vi "Execute Add Actor Message.vi"(6 "Mouse Position":T1 caption="鼠标位置", 8 "User VI Ref":refnum<vi> caption="用户VI引用", 9 "Menu Item Tag Suffix":string caption="菜单项标签后缀", 10 "Remaining Items":refnum<vi>[](array[refnum]) caption="剩余项", 11 "Affected Items":T2 caption="受影响的项") -> (0 "Fail transaction?":bool caption="操作失败？")   [LabVIEW 2020]
doc: "该VI属于修改LabVIEW快捷菜单部分。这是用户选择快捷菜单时调用的执行VI。该VI执行选中菜单项的操作。"
uses:
  Add Actor Message.ctl
  <vilib>/Utility/miscctls.llb/LVPositionTypeDef.ctl
panel:
  # "除“受影响的项”之外，前面板上的其他所有控件都已锁定，以防被意外编辑。修改控件名称或类型，而不是“受影响的项”簇的元素将使VI无法作为菜单插件使用。\n\n请参考每个控件的即时帮助了解其用法。"
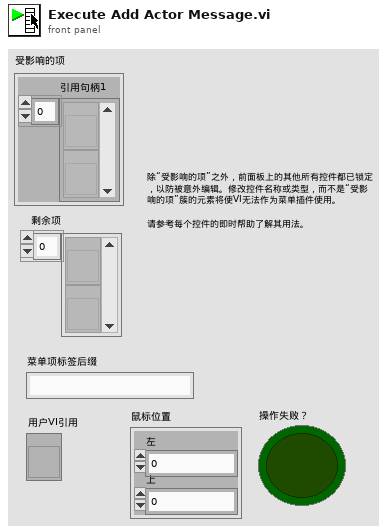
[diagram p1: front panel]
types:
  T1 = typedef "LVPositionTypeDef.ctl" = cluster{"Left":i32, "Top":i32}
  T2 = typedef "Add Actor Message.ctl" = cluster{"GObj":refnum<vi>[]}
  T3 = typedef "LVRectTypeDef.ctl" = cluster{"Left":i16, "Top":i16, "Right":i16, "Bottom":i16}
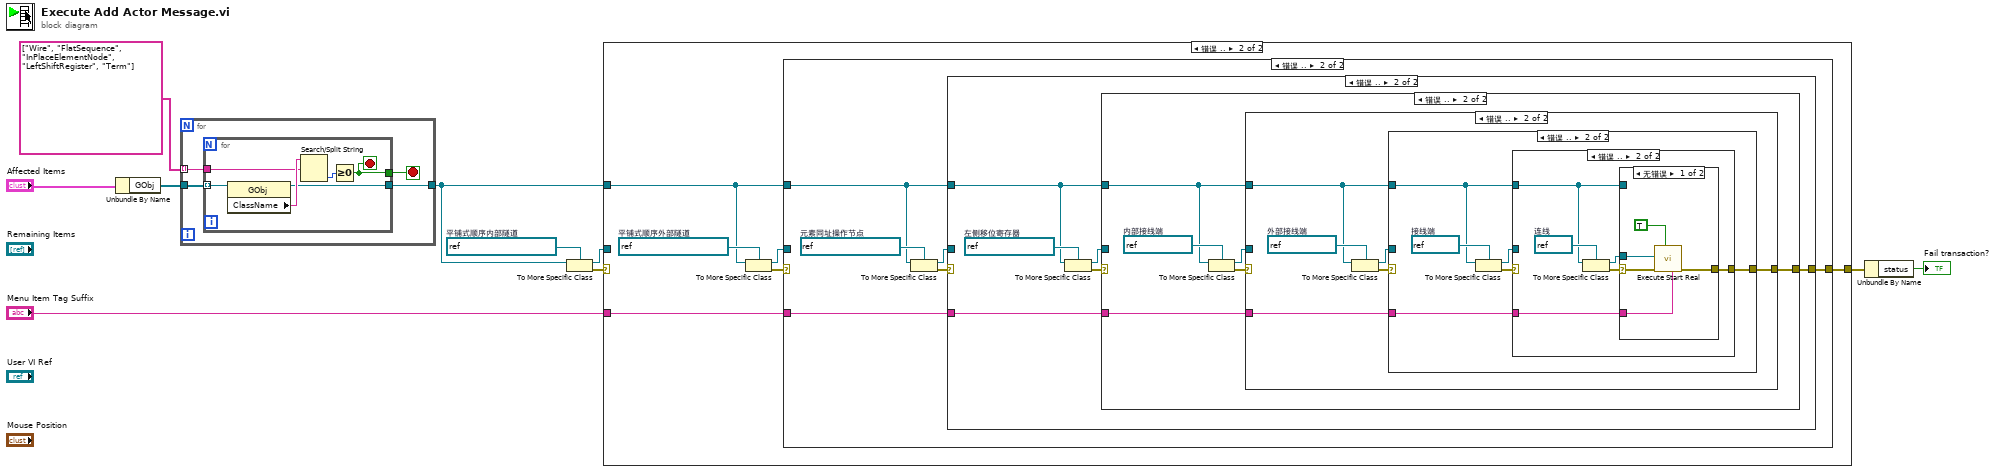
[diagram p0: block diagram]
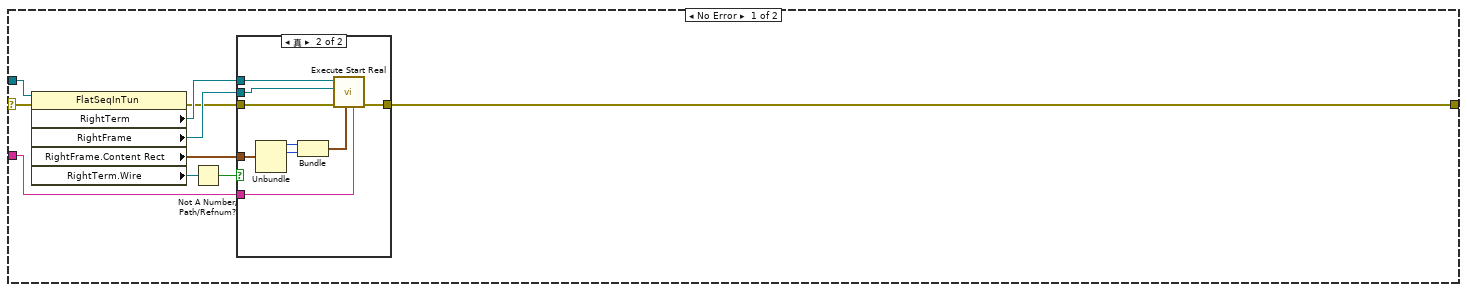
[diagram p2: hidden frame]
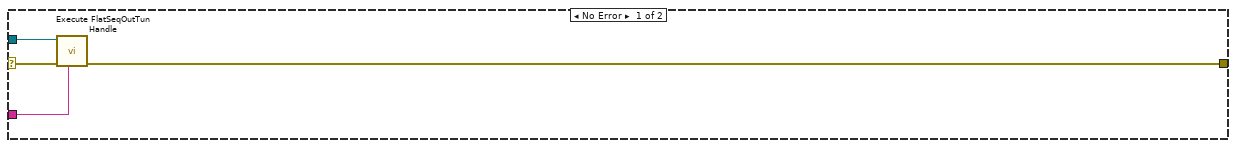
[diagram p4: hidden frame]
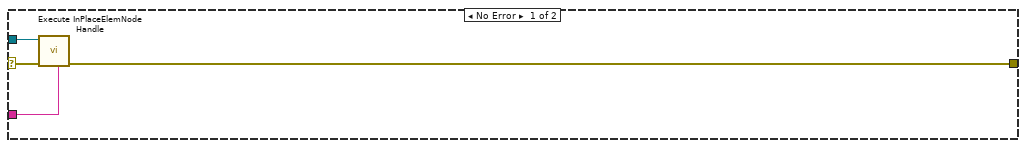
[diagram p5: hidden frame]
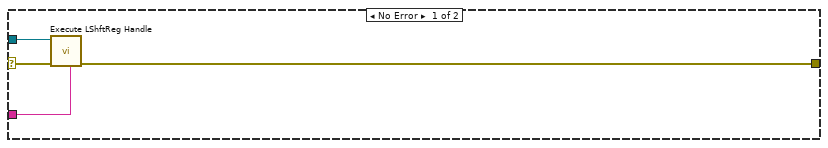
[diagram p6: hidden frame]
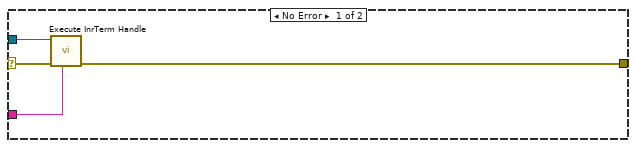
[diagram p7: hidden frame]
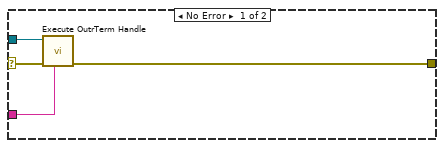
[diagram p8: hidden frame]
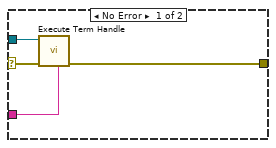
[diagram p9: hidden frame]
diagram:
  w6 = refnum<vi> refnum  # 平铺式顺序内部隧道
  n1 = Unbundle By Name("Affected Items") -> ("GObj"=w9:refnum<vi>[])
  n2 = for {
    tunnel: w9 -> [w14]
    tunnel: string[] ["Wire", "FlatSequence", "InPlaceElementNode", "LeftShiftRegister", "Term"] ("可处理类型") -> [w13] mode=indexing
    tunnel: [w11] -> w5
    stop <- w12 stop-if-true
    n3 = for {
      tunnel: w14 -> [w20] mode=indexing
      tunnel: w13 -> [w18]
      tunnel: [w16] -> w12
      tunnel: [w15] -> w11
      stop <- w16 stop-if-true
      n4 = property class="GObj"(reference=w20) -> (reference out=w15:refnum<vi>, "ClassName"=w19:string)  [unwired: 1 in, 1 out]
      n5 = Search/Split String(string=w19, search string/char (-)=w18) -> (offset of match=w17:i32)  [unwired: 1 in, 2 out]
      n6 = Greater Or Equal To 0?(x=w17) -> (x >= 0?=w16:bool)
    }
  }
  n7 = To More Specific Class(target class=w6, reference=w5) -> (specific class reference=w3:refnum<vi>, error out=w4:errorcluster)  [unwired: 1 in]
  n8 = case shown="错误 .." w4 {
    selector: w4 -> [w24 _]
    tunnel: "Menu Item Tag Suffix" -> [w22 w46]
    tunnel: w5 -> [_ w43]
    tunnel: w3 -> [w28 _]
    tunnel: [w21 w41] -> w2
    frame No Error {
      n9 = property class="FlatSeqInTun"(reference=w28, error in=w24) -> (error out=w23:errorcluster, "RightTerm"=w29:refnum<vi>, "RightFrame"=w30:refnum<vi>, "RightFrame.Content Rect"=w27:T3, "RightTerm.Wire"=w26:refnum<vi>)  [unwired: 1 out]
      n10 = Not A Number/Path/Refnum?(number/path/refnum=w26) -> (NaN/Path/Refnum?=w25:bool)
      n11 = case shown="真" w25 {
        tunnel: w30 -> [_ w40]
        tunnel: w29 -> [_ w39]
        tunnel: w27 -> [_ w36]
        tunnel: w23 -> [w31 w34]
        tunnel: [w31 w33] -> w21
        tunnel: w22 -> [_ w32]
        frame False {
        }
        frame True {
          n12 = Unbundle(w36) -> ("Left"=w38:i16, "Top"=w37:i16)  [unwired: 2 out]
          n13 = Bundle("Left"=w38, "Top"=w37) -> (w35:cluster{"Left":i16, "Top":i16})  [unwired: 1 in]
          n14 = call "Execute Start Real.vi"("Menu Item Tag Suffix"=w32, "相对位置原点"=w35, "错误输入（无错误）"=w34, "所有者引用句柄"=w40, "接线端输入"=w39) -> ("错误输出"=w33:errorcluster)  [unwired: 6 in]
        }
      }
    }
    frame Error {
      w45 = refnum<vi> refnum  # 平铺式顺序外部隧道
      n15 = To More Specific Class(target class=w45, reference=w43) -> (specific class reference=w42:refnum<vi>, error out=w44:errorcluster)  [unwired: 1 in]
      n16 = case shown="错误 .." w44 {
        selector: w44 -> [w48 _]
        tunnel: w46 -> [w47 w56]
        tunnel: w43 -> [_ w52]
        tunnel: w42 -> [w50 _]
        tunnel: [w49 w51] -> w41
        frame No Error {
          n17 = call "Execute FlatSeqOutTun Handle.vi"("Menu Item Tag Suffix"=w47, "错误输入（无错误）"=w48, "平铺式顺序外部隧道输入"=w50) -> ("错误输出"=w49:errorcluster)  [unwired: 8 in]
        }
        frame Error {
          w55 = refnum<vi> refnum  # 元素同址操作节点
          n18 = To More Specific Class(target class=w55, reference=w52) -> (specific class reference=w53:refnum<vi>, error out=w54:errorcluster)  [unwired: 1 in]
          n19 = case shown="错误 .." w54 {
            selector: w54 -> [w59 _]
            tunnel: w56 -> [w57 w66]
            tunnel: w52 -> [_ w62]
            tunnel: w53 -> [w60 _]
            tunnel: [w58 w61] -> w51
            frame No Error {
              n20 = call "Execute InPlaceElemNode Handle.vi"("Menu Item Tag Suffix"=w57, "错误输入（无错误）"=w59, "元素同址操作节点输入"=w60) -> ("错误输出"=w58:errorcluster)  [unwired: 8 in]
            }
            frame Error {
              w63 = refnum<vi> refnum  # 左侧移位寄存器
              n21 = To More Specific Class(target class=w63, reference=w62) -> (specific class reference=w64:refnum<vi>, error out=w65:errorcluster)  [unwired: 1 in]
              n22 = case shown="错误 .." w65 {
                selector: w65 -> [w69 _]
                tunnel: w66 -> [w68 w76]
                tunnel: w62 -> [_ w72]
                tunnel: w64 -> [w70 _]
                tunnel: [w67 w71] -> w61
                frame No Error {
                  n23 = call "Execute LShftReg Handle.vi"("Menu Item Tag Suffix"=w68, "错误输入（无错误）"=w69, "左侧移位寄存器输入"=w70) -> ("错误输出"=w67:errorcluster)  [unwired: 8 in]
                }
                frame Error {
                  w73 = refnum<vi> refnum  # 内部接线端
                  n24 = To More Specific Class(target class=w73, reference=w72) -> (specific class reference=w74:refnum<vi>, error out=w75:errorcluster)  [unwired: 1 in]
                  n25 = case shown="错误 .." w75 {
                    selector: w75 -> [w79 _]
                    tunnel: w72 -> [_ w85]
                    tunnel: w76 -> [w78 w82]
                    tunnel: w74 -> [w80 _]
                    tunnel: [w77 w81] -> w71
                    frame No Error {
                      n26 = call "Execute InrTerm Handle.vi"("Menu Item Tag Suffix"=w78, "错误输入（无错误）"=w79, "内部接线端输入"=w80) -> ("错误输出"=w77:errorcluster)  [unwired: 8 in]
                    }
                    frame Error {
                      w86 = refnum<vi> refnum  # 外部接线端
                      n27 = To More Specific Class(target class=w86, reference=w85) -> (specific class reference=w83:refnum<vi>, error out=w84:errorcluster)  [unwired: 1 in]
                      n28 = case shown="错误 .." w84 {
                        selector: w84 -> [w88 _]
                        tunnel: w85 -> [_ w94]
                        tunnel: w83 -> [w90 _]
                        tunnel: w82 -> [w89 w92]
                        tunnel: [w87 w91] -> w81
                        frame No Error {
                          n29 = call "Execute OutrTerm Handle.vi"("Menu Item Tag Suffix"=w89, "错误输入（无错误）"=w88, "外部接线端输入"=w90) -> ("错误输出"=w87:errorcluster)  [unwired: 8 in]
                        }
                        frame Error {
                          w96 = refnum<vi> refnum  # 接线端
                          n30 = To More Specific Class(target class=w96, reference=w94) -> (specific class reference=w93:refnum<vi>, error out=w95:errorcluster)  [unwired: 1 in]
                          n31 = case shown="错误 .." w95 {
                            selector: w95 -> [w100 _]
                            tunnel: w94 -> [_ w103]
                            tunnel: w93 -> [w99 _]
                            tunnel: w92 -> [w98 w102]
                            tunnel: [w97 w101] -> w91
                            frame No Error {
                              n32 = call "Execute Term Handle.vi"("Menu Item Tag Suffix"=w98, "错误输入（无错误）"=w100, "接线端输入"=w99) -> ("错误输出"=w97:errorcluster)  [unwired: 8 in]
                            }
                            frame Error {
                              w106 = refnum<vi> refnum  # 连线
                              n33 = To More Specific Class(target class=w106, reference=w103) -> (specific class reference=w105:refnum<vi>, error out=w104:errorcluster)  [unwired: 1 in]
                              n34 = case shown="无错误" w104 {
                                selector: w104 -> [w111 w112]
                                tunnel: w105 -> [w110 _]
                                tunnel: w103 -> [_ _]
                                tunnel: w102 -> [w108 _]
                                tunnel: [w107 w112] -> w101
                                frame No Error {
                                n35 = call "Execute Start Real.vi"("Menu Item Tag Suffix"=w108, "Insert?"=TRUE, "错误输入（无错误）"=w111, "所有者引用句柄"=w110) -> ("错误输出"=w107:errorcluster)  [unwired: 7 in]
                                }
                                frame Error {
                                }
                              }
                            }
                          }
                        }
                      }
                    }
                  }
                }
              }
            }
          }
        }
      }
    }
  }
  n36 = Unbundle By Name(w2) -> ("status"=→"Fail transaction?":bool)
